vi "execute.vi"(8 "error in (no error)":errorcluster, 9 "trajectory resonance in":refnum<class "GenericComponent.lvclass">, 10 "imaging mode in":refnum<class "GenericComponent.lvclass">, 11 "AdapterAK101022ImagingModeToTrajectory in":refnum<class "AdapterAK101022ImagingModeToTrajectory.lvclass">) -> (0 "error out":errorcluster, 1 "trajectory resonance out":refnum<class "GenericComponent.lvclass">, 2 "imaging mode out":refnum<class "GenericComponent.lvclass">, 3 "AdapterAK101022ImagingModeToTrajectory out":refnum<class "AdapterAK101022ImagingModeToTrajectory.lvclass">)   [LabVIEW 2010, in "AdapterAK101022ImagingModeToTrajectory.lvclass"]
uses:
  AdapterAK101022ImagingModeToTrajectory.lvclass
  common/classes/GenericComponent/GenericComponent/GenericComponent.lvclass
  ImagingMode/ImagingModeDL090130Frame/ImagingModeDL090130Frame/ImagingModeDL090130Frame.lvclass
  Trajectory/TrajectoryAK101022Resonance/TrajectoryAK101022Resonance/TrajectoryAK101022Resonance.lvclass
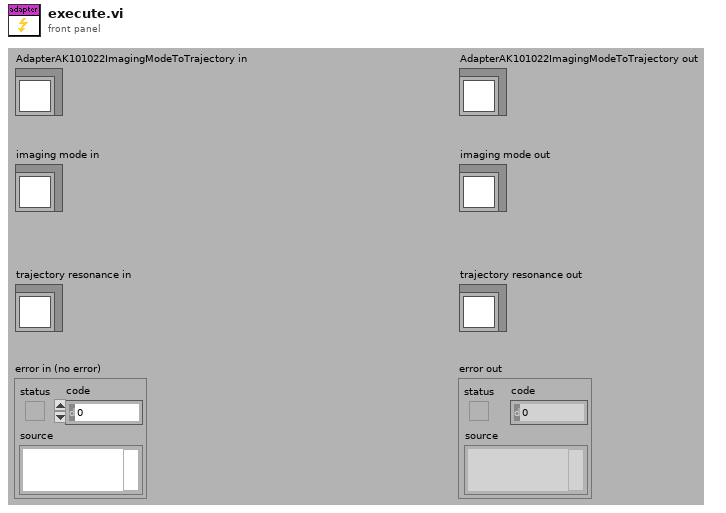
[diagram p1: front panel]
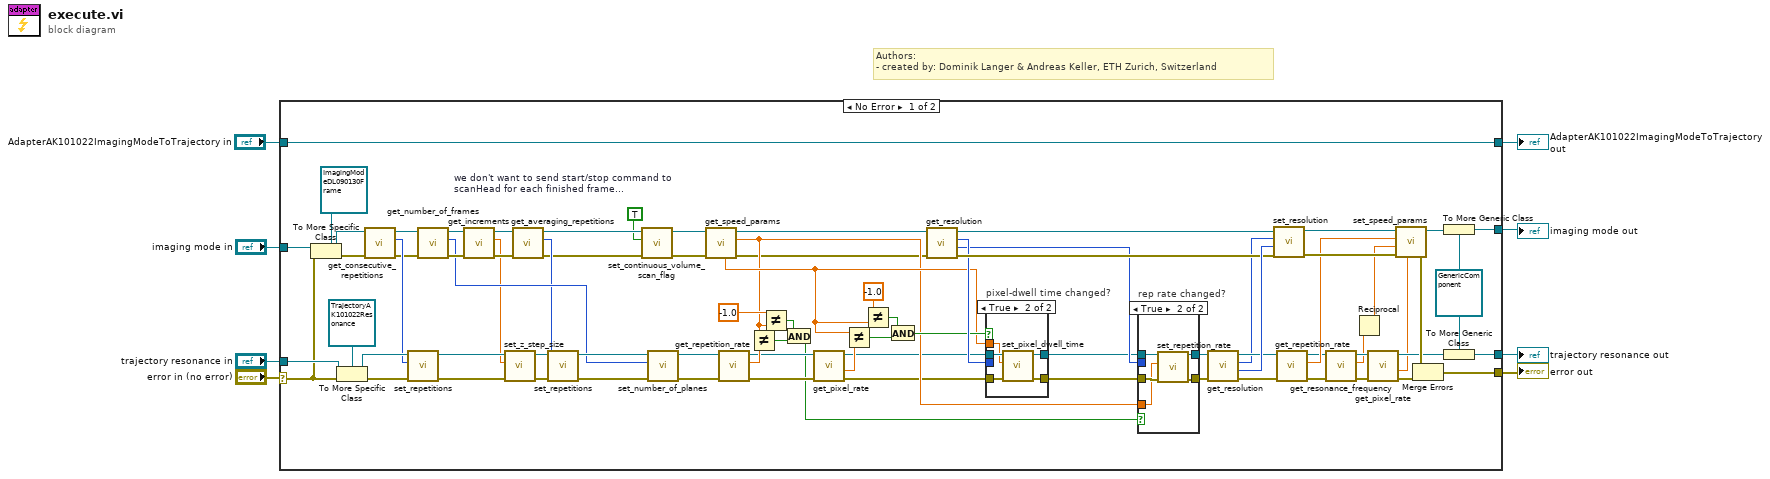
[diagram p0: block diagram]
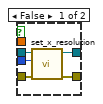
[diagram p2: hidden frame]
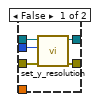
[diagram p3: hidden frame]
diagram:
  # "Authors: \n- created by: Dominik Langer & Andreas Keller, ETH Zurich, Switzerland"
  n1 = case shown="No Error" "error in (no error)" {
    selector: "error in (no error)" -> [w81 w110]
    tunnel: "AdapterAK101022ImagingModeToTrajectory in" -> [w89 w113]
    tunnel: [w89 w113] -> w6
    tunnel: [w83 w112] -> w4
    tunnel: "imaging mode in" -> [w86 w112]
    tunnel: [w84 w111] -> w2
    tunnel: "trajectory resonance in" -> [w88 w111]
    tunnel: [w73 w110] -> w1
    frame No Error {
      w9 = TRUE  # we don't want to send start/stop command to scanHead for each finished frame...
      w82 = refnum<class "GenericComponent.lvclass"> refnum ("GenericComponent.lvclass")
      n2 = To More Specific Class(target class=refnum<class "ImagingModeDL090130Frame.lvclass"> refnum ("DL090130FrameScanMode.lvclass"), reference=w86, error in=w81) -> (specific class reference=w36:refnum<class "ImagingModeDL090130Frame.lvclass">, error out=w37:errorcluster)
      n3 = To More Specific Class(target class=refnum<class "TrajectoryAK101022Resonance.lvclass"> refnum ("TrajectoryAK101022Resonance.lvclass"), reference=w88, error in=w81) -> (specific class reference=w35:refnum<class "TrajectoryAK101022Resonance.lvclass">, error out=w33:errorcluster)
      n4 = call-dynamic "get_consecutive_repetitions.vi"("error in (no error)"=w37, "ImagingModeDL090130Frame in"=w36) -> ("error out"=w28:errorcluster, "number of consecutive repetitions"=w34:i32, "ImagingModeDL090130Frame out"=w25:refnum<class "ImagingModeDL090130Frame.lvclass">)  [unwired: 7 in]
      n5 = call-dynamic "set_repetitions.vi"("error in (no error)"=w33, "repetitions per frame"=w34, "TrajectoryAK101022Resonance in"=w35) -> ("error out"=w22:errorcluster, "TrajectoryAK101022Resonance out"=w18:refnum<class "TrajectoryAK101022Resonance.lvclass">)  [unwired: 7 in]
      n6 = call-dynamic "get_number_of_frames.vi"("error in (no error)"=w28, "ImagingModeDL090130Frame in"=w25) -> ("error out"=w30:errorcluster, "number of frames"=w16:i32, "ImagingModeDL090130Frame out"=w27:refnum<class "ImagingModeDL090130Frame.lvclass">)  [unwired: 7 in]
      n7 = call-dynamic "get_increments.vi"("error in (no error)"=w30, "ImagingModeDL090130Frame in"=w27) -> ("error out"=w29:errorcluster, "step size"=w15:dbl[unit], "ImagingModeDL090130Frame out"=w26:refnum<class "ImagingModeDL090130Frame.lvclass">)  [unwired: 7 in]
      n8 = call-dynamic "set_z_step_size.vi"("error in (no error)"=w22, "z step size"=w15, "TrajectoryAK101022Resonance in"=w18) -> ("error out"=w24:errorcluster, "TrajectoryAK101022Resonance out"=w20:refnum<class "TrajectoryAK101022Resonance.lvclass">)  [unwired: 7 in]
      n9 = call-dynamic "get_averaging_repetitions.vi"("error in (no error)"=w29, "ImagingModeDL090130Frame in"=w26) -> ("error out"=w12:errorcluster, "averaging repetitions"=w14:i32, "ImagingModeDL090130Frame out"=w13:refnum<class "ImagingModeDL090130Frame.lvclass">)  [unwired: 7 in]
      n10 = call-dynamic "set_repetitions.vi"("error in (no error)"=w24, "repetitions per frame"=w14, "TrajectoryAK101022Resonance in"=w20) -> ("error out"=w23:errorcluster, "TrajectoryAK101022Resonance out"=w19:refnum<class "TrajectoryAK101022Resonance.lvclass">)  [unwired: 7 in]
      n11 = call "set_continuous_volume_scan_flag.vi"("error in (no error)"=w12, "continuous volume scan?"=w9, "ImagingModeDL090130Frame in"=w13) -> ("error out"=w11:errorcluster, "ImagingModeDL090130Frame out"=w10:refnum<class "ImagingModeDL090130Frame.lvclass">)  [unwired: 7 in]
      n12 = call-dynamic "set_number_of_planes.vi"("error in (no error)"=w23, "Number of planes"=w16, "TrajectoryAK101022Resonance in"=w19) -> ("error out"=w21:errorcluster, "TrajectoryAK101022Resonance out"=w17:refnum<class "TrajectoryAK101022Resonance.lvclass">)  [unwired: 7 in]
      n13 = call-dynamic "get_speed_params.vi"("error in (no error)"=w11, "ImagingModeDL090130Frame in"=w10) -> ("error out"=w39:errorcluster, "frame rate"=w40:dbl[unit], "ImagingModeDL090130Frame out"=w38:refnum<class "ImagingModeDL090130Frame.lvclass">, "pixel dwell time"=w41:dbl[unit])  [unwired: 4 in, 2 out]
      n14 = call-dynamic "get_repetition_rate.vi"("error in (no error)"=w21, "GenericTrajectory in"=w17) -> ("error out"=w54:errorcluster, "repetition rate"=w70:dbl[unit], "GenericTrajectory out"=w55:refnum<class "TrajectoryAK101022Resonance.lvclass">)  [unwired: 7 in]
      n15 = Not Equal?(x=w40, y=w70) -> (x != y?=w49:bool)
      n16 = Not Equal?(x=dbl[unit] -1.0, y=w40) -> (x != y?=w48:bool)
      n17 = And(x=w48, y=w49) -> (x .and. y?=w42:bool)
      n18 = call-dynamic "get_pixel_rate.vi"("error in (no error)"=w54, "TrajectoryAK101022Resonance in"=w55) -> ("error out"=w32:errorcluster, "pixel dwell time"=w53:dbl[unit], "TrajectoryAK101022Resonance out"=w31:refnum<class "TrajectoryAK101022Resonance.lvclass">)  [unwired: 6 in, 1 out]
      n19 = Not Equal?(x=w41, y=w53) -> (x != y?=w46:bool)
      n20 = Not Equal?(x=dbl[unit] -1.0, y=w41) -> (x != y?=w45:bool)
      n21 = And(x=w45, y=w46) -> (x .and. y?=w44:bool)
      n22 = call-dynamic "get_resolution.vi"("error in (no error)"=w39, "ImagingModeDL090130Frame in"=w38) -> ("error out"=w79:errorcluster, "y resolution"=w76:i32, "x resolution"=w78:i32, "ImagingModeDL090130Frame out"=w77:refnum<class "ImagingModeDL090130Frame.lvclass">)  [unwired: 6 in]
      n23 = case "pixel-dwell time changed?" shown="True" w44 {
        tunnel: w78 -> [w94 _]
        tunnel: w31 -> [w93 w96]
        tunnel: w32 -> [w92 w99]
        tunnel: [w91 w98] -> w51
        tunnel: [w90 w97] -> w50
        tunnel: w41 -> [_ w95]
        frame False {
          n24 = call-dynamic "set_x_resolution.vi"("error in (no error)"=w92, "x resolution"=w94, "TrajectoryAK101022Resonance in"=w93) -> ("error out"=w91:errorcluster, "TrajectoryAK101022Resonance out"=w90:refnum<class "TrajectoryAK101022Resonance.lvclass">)  [unwired: 7 in]
        }
        frame True {
          n25 = call-dynamic "set_pixel_dwell_time.vi"("error in (no error)"=w99, "pixel-dwell time"=w95, "TrajectoryAK101022Resonance in"=w96) -> ("error out"=w98:errorcluster, "TrajectoryAK101022Resonance out"=w97:refnum<class "TrajectoryAK101022Resonance.lvclass">)  [unwired: 7 in]
        }
      }
      n26 = case "rep rate changed?" shown="True" w42 {
        tunnel: w51 -> [w104 w107]
        tunnel: w50 -> [w103 w108]
        tunnel: w76 -> [w102 _]
        tunnel: [w101 w106] -> w72
        tunnel: [w100 w109] -> w71
        tunnel: w40 -> [_ w105]
        frame False {
          n27 = call-dynamic "set_y_resolution.vi"("error in (no error)"=w104, "y resolution"=w102, "TrajectoryAK101022Resonance in"=w103) -> ("error out"=w101:errorcluster, "TrajectoryAK101022Resonance out"=w100:refnum<class "TrajectoryAK101022Resonance.lvclass">)  [unwired: 7 in]
        }
        frame True {
          n28 = call-dynamic "set_repetition_rate.vi"("error in (no error)"=w107, "repetition rate"=w105, "TrajectoryAK101022Resonance in"=w108) -> ("error out"=w106:errorcluster, "TrajectoryAK101022Resonance out"=w109:refnum<class "TrajectoryAK101022Resonance.lvclass">)  [unwired: 7 in]
        }
      }
      n29 = call-dynamic "get_resolution.vi"("error in (no error)"=w72, "TrajectoryAK101022Resonance in"=w71) -> ("error out"=w75:errorcluster, "y resolution"=w80:i32, "x resolution"=w52:i32, "TrajectoryAK101022Resonance out"=w74:refnum<class "TrajectoryAK101022Resonance.lvclass">)  [unwired: 6 in]
      n30 = call-dynamic "set_resolution.vi"("error in (no error)"=w79, "y"=w80, "x"=w52, "ImagingModeDL090130Frame in"=w77) -> ("error out"=w69:errorcluster, "ImagingModeDL090130Frame out"=w67:refnum<class "ImagingModeDL090130Frame.lvclass">)  [unwired: 6 in]
      n31 = call-dynamic "get_repetition_rate.vi"("error in (no error)"=w75, "GenericTrajectory in"=w74) -> ("error out"=w61:errorcluster, "repetition rate"=w68:dbl[unit], "GenericTrajectory out"=w59:refnum<class "TrajectoryAK101022Resonance.lvclass">)  [unwired: 7 in]
      n32 = call-dynamic "get_resonance_frequency.vi"("error in (no error)"=w61, "TrajectoryAK101022Resonance in"=w59) -> ("error out"=w60:errorcluster, "resonance frequency"=w57:dbl[unit], "TrajectoryAK101022Resonance out"=w58:refnum<class "TrajectoryAK101022Resonance.lvclass">)  [unwired: 7 in]
      n33 = Reciprocal(x=w57) -> (1/x=w56:dbl[unit])
      n34 = call-dynamic "get_pixel_rate.vi"("error in (no error)"=w60, "TrajectoryAK101022Resonance in"=w58) -> ("error out"=w64:errorcluster, "pixel dwell time"=w62:dbl[unit], "TrajectoryAK101022Resonance out"=w63:refnum<class "TrajectoryAK101022Resonance.lvclass">)  [unwired: 6 in, 1 out]
      n35 = call-dynamic "set_speed_params.vi"("pixel-dwell time"=w62, "error in (no error)"=w69, "line-scan time"=w56, "frame rate"=w68, "ImagingModeDL090130Frame in"=w67) -> ("error out"=w65:errorcluster, "ImagingModeDL090130Frame out"=w66:refnum<class "ImagingModeDL090130Frame.lvclass">)  [unwired: 5 in]
      n36 = Merge Errors(w65, w64) -> (w73:errorcluster)
      n37 = To More Generic Class(target class=w82, reference=w66) -> (generic class reference=w83:refnum<class "GenericComponent.lvclass">)
      n38 = To More Generic Class(target class=w82, reference=w63) -> (generic class reference=w84:refnum<class "GenericComponent.lvclass">)
    }
    frame Error {
    }
  }
  "error out" <- w1
  "AdapterAK101022ImagingModeToTrajectory out" <- w6
  "imaging mode out" <- w4
  "trajectory resonance out" <- w2
